vi "Write Engine Cluster.vi"(8 "error in (no error)":errorcluster, 10 "Engine Cluster":T1, 11 "Abstract Engine in":refnum<class "Abstract Engine.lvclass">) -> (0 "error out":errorcluster, 3 "Abstract Engine out":refnum<class "Abstract Engine.lvclass">)   [LabVIEW 2025, in "Abstract Engine.lvlib" / "Abstract Engine.lvclass"]
uses:
  Abstract Engine.lvclass
  Engine Cluster.ctl
  Users/Public/Documents/Sandia National Labs/TSS Plugin/Interface.lvlibp/Analog Input/Channel.ctl
  Abstract Engine.lvclass/Abstract Engine.ctl
  Users/Public/Documents/Sandia National Labs/TSS Plugin/Interface.lvlibp/Analog Input/AI.lvclass
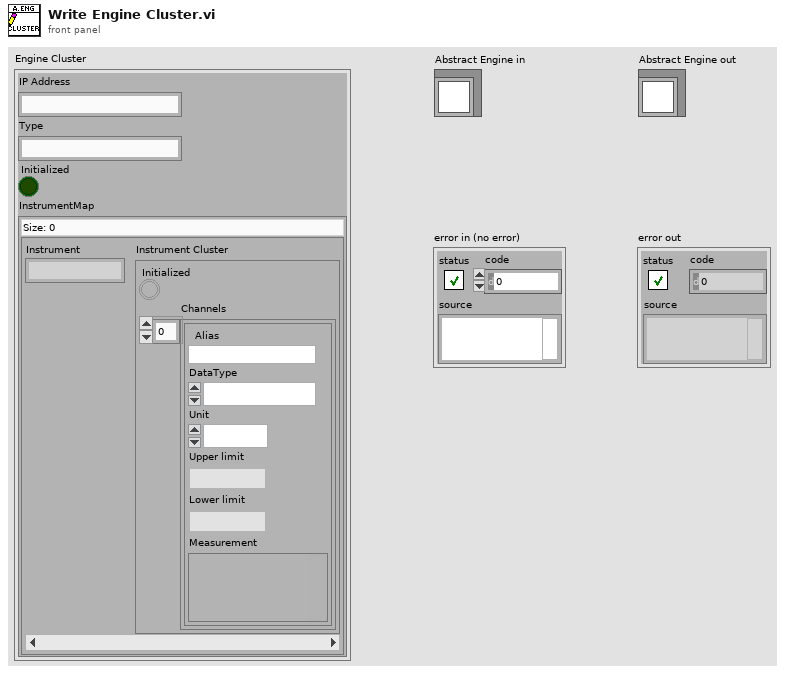
[diagram p1: front panel]
types:
  T1 = typedef "Abstract Engine.lvlib/Abstract Engine.lvclass/Engine Cluster.ctl" = cluster{"IP Address":string, "Type":string, "Initialized":bool, "InstrumentMap":map{string, cluster{"Initialized":bool, "Channels":T2[]}}}
  T2 = typedef "Interface.lvlibp/AI.lvclass/Channel.ctl" = cluster{"Alias":string, "DataType":enum16{"Anaolg Input", "Waveform"}, "Unit":enum16{"---", "V", "A", "Ohm", "Hz", "uF", "degC", "deg"}, "Upper limit":dbl, "Lower limit":dbl, "Measurement":variant}
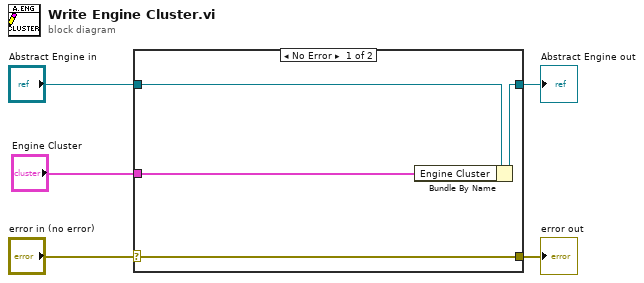
[diagram p0: block diagram]
diagram:
  n1 = case shown="No Error" "error in (no error)" {
    selector: "error in (no error)" -> [w9 w10]
    tunnel: [w9 w10] -> w4
    tunnel: [w7 w11] -> w2
    tunnel: "Abstract Engine in" -> [w8 w11]
    tunnel: "Engine Cluster" -> [w6 _]
    frame No Error {
      n2 = Bundle By Name(cluster=w8, "Engine Cluster"=w6) -> (w7:refnum<class "Abstract Engine.lvclass">)
    }
    frame Error {
    }
  }
  "error out" <- w4
  "Abstract Engine out" <- w2
